vi "PatternPath.vi"() -> (0 "数据文件":path, 1 "CameraData":path, 2 "PatternPath":path, 3 "料号":path, 4 "快捷菜单":path, 5 "SIM2.0":path caption="应用程序目录")   [LabVIEW 2015]
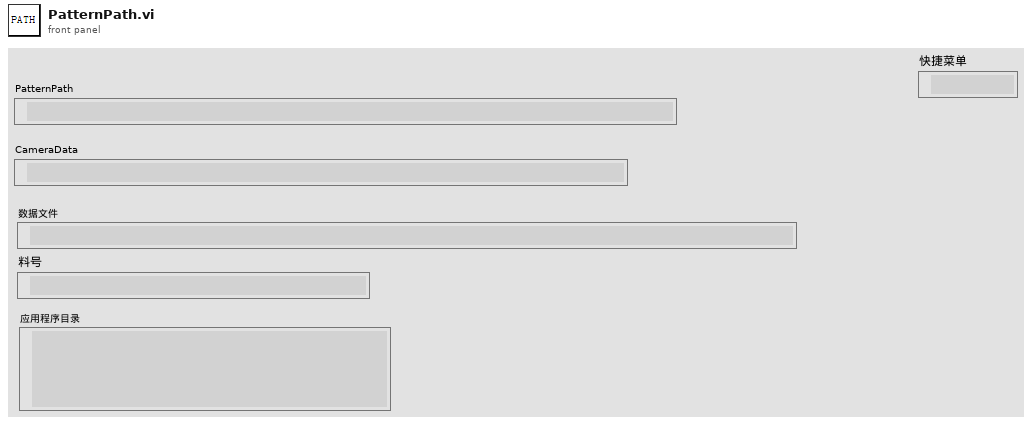
[diagram p1: front panel]
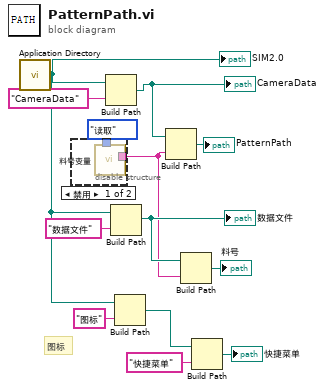
[diagram p0: block diagram]
diagram:
  # "图标"
  n1 = call <vilib>:"Application Directory.vi"() -> ("Application Directory"=w5:path)
  "SIM2.0" <- w5
  n2 = disable-structure shown="禁用" {
    disable-tunnel: enum16{"读取", "写入"}."读取" ("枚举") -> [w15 _]
    disable-tunnel: [w14 _] -> w6
    frame Disabled {
      n3 = call "料号变量.vi"("枚举"=w15) -> ("料号Out"=w14:string)  [unwired: 10 in]
    }
    frame Enabled {
    }
  }
  n4 = Build Path(base path=w5, name or relative path="CameraData" ("名称或相对路径")) -> (appended path=w11:path)
  "CameraData" <- w11
  n5 = Build Path(base path=w5, name or relative path="数据文件" ("名称或相对路径")) -> (appended path=w8:path)
  "数据文件" <- w8
  n6 = Build Path(base path=w5, name or relative path="图标" ("名称或相对路径")) -> (appended path=w3:path)
  n7 = Build Path(base path=w11, name or relative path=w6) -> (appended path=→"PatternPath":path)
  n8 = Build Path(base path=w8, name or relative path=w6) -> (appended path=→"料号":path)
  n9 = Build Path(base path=w3, name or relative path="快捷菜单" ("名称或相对路径")) -> (appended path=→"快捷菜单":path)
